vi "create.vi"(8 "error in (no error)":errorcluster, 10 "Cluster.Array":bool[](array[boolean])=[FALSE], 11 "tempy in":refnum<class "array-in-a-cluster.lvclass">) -> (0 "error out":errorcluster, 3 "tempy out":refnum<class "array-in-a-cluster.lvclass">)   [LabVIEW 2020, in "TEST - JKI JSON Object Serialization.lvlib" / "array-in-a-cluster.lvclass"]
uses:
  array-in-a-cluster.lvclass
  array-in-a-cluster.lvclass/array-in-a-cluster.ctl
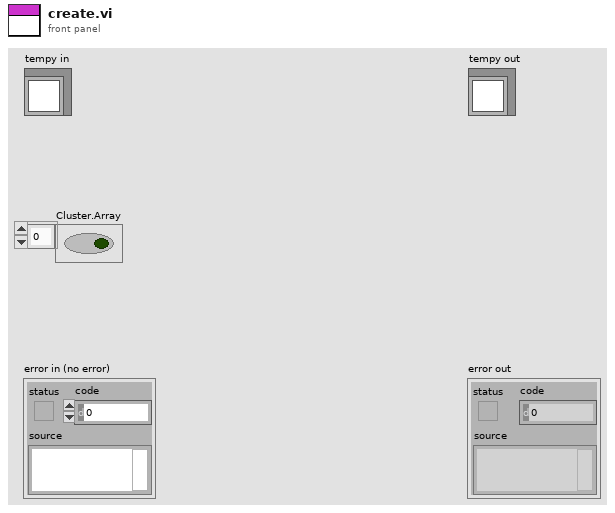
[diagram p1: front panel]
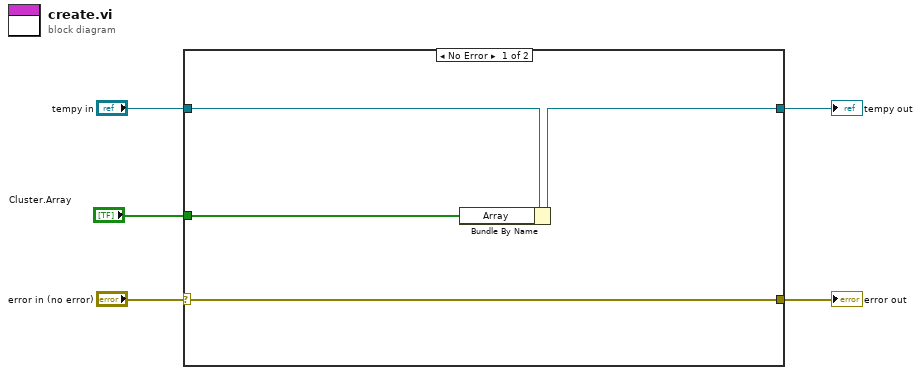
[diagram p0: block diagram]
diagram:
  n1 = case shown="No Error" "error in (no error)" {
    selector: "error in (no error)" -> [w9 w11]
    tunnel: [w9 w11] -> w4
    tunnel: [w8 w10] -> w2
    tunnel: "tempy in" -> [w7 w10]
    tunnel: "Cluster.Array" -> [w6 _]
    frame No Error {
      n2 = Bundle By Name(cluster=w7, "Array"=w6) -> (w8:refnum<class "array-in-a-cluster.lvclass">)
    }
    frame Error {
    }
  }
  "error out" <- w4
  "tempy out" <- w2
